vi "pid.vi"(7 "reset":bool, 8 "PID gains":T1, 9 "Enable motors":bool, 10 "Speed":cluster{"Left":dbl, "right":dbl}, 11 "Refnum in":refnum<k20>) -> (1 "output Speed":cluster{dbl, dbl}, 3 "Refnum out":refnum<k20>, 4 "dt out (s)":dbl format="%.3f")   [LabVIEW 2019]
uses:
  <vilib>/addons/control/pid/pid.llb/PID (DBL).vi
  <vilib>/Utility/error.llb/Error Cluster From Error Code.vi
  <vilib>/rvi/errors/niLvFpgaAdjustHostInterfaceError.vi
  <vilib>/rvi/interface/nirviReadWriteControl/nirviReadWriteControl.xnode
  NiFpgaLv.dll
  <vilib>/rvi/interface/Simulation/niFpgaSimulationCallBeginRW.vi
  <vilib>/addons/control/pid/NI_PID_pid.lvlib
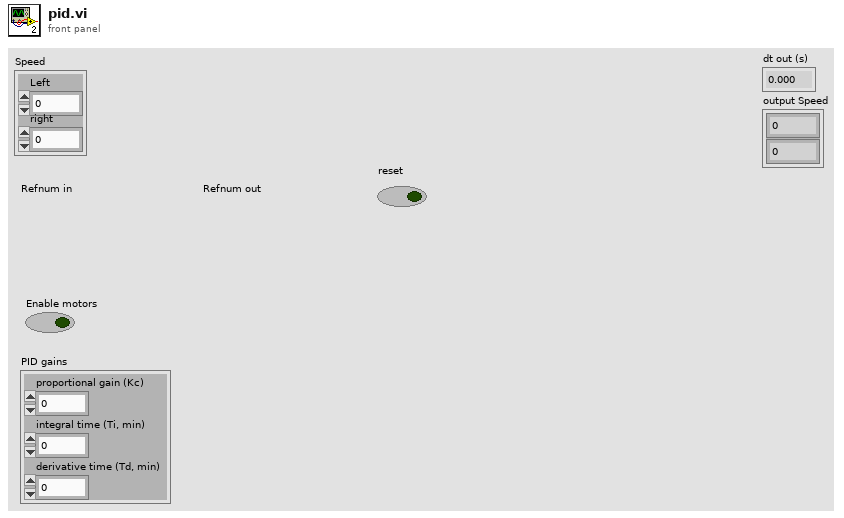
[diagram p1: front panel]
types:
  T1 = cluster{"proportional gain (Kc)":dbl, "integral time (Ti, min)":dbl, "derivative time (Td, min)":dbl}
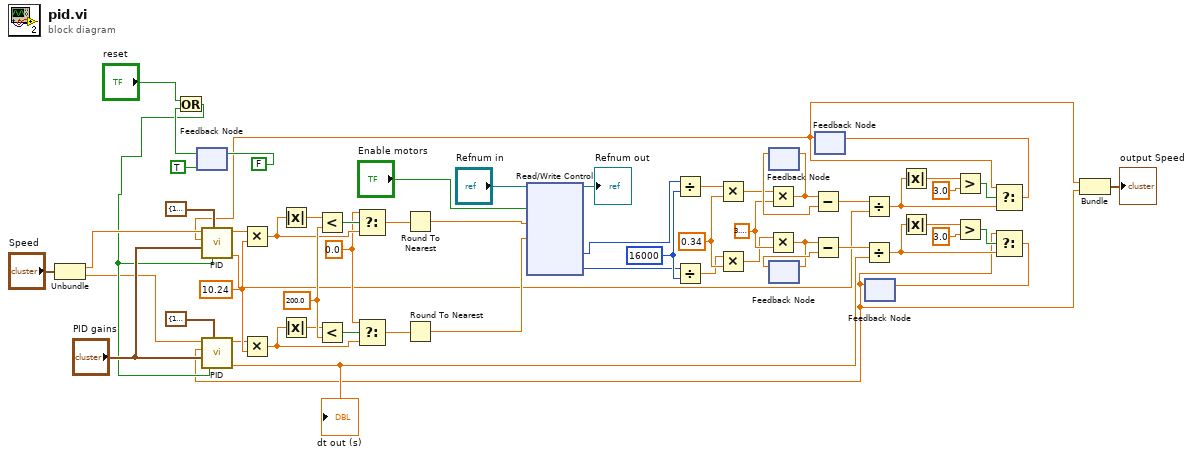
[diagram p0: block diagram]
diagram:
  w54 = 200.0 ("y")
  w47 = 0.0 ("t")
  w44 = 10.24 ("y")
  w26 = 3.141592653589793
  w23 = 0.34
  w20 = i64 16000 ("y")
  n1 = Unbundle("Speed") -> ("Left"=w9:dbl, "right"=w2:dbl)
  n2 = feedback #1(TRUE) -> (w5:bool)
  n3 = Or(x="reset", y=w5) -> (x .or. y?=w3:bool)
  n4 = feedback-in #1(FALSE) -> ()
  n5 = feedback #2() -> (w30:dbl)  [unwired: 1 in]
  n6 = feedback #3() -> (w28:dbl)  [unwired: 1 in]
  n7 = feedback #4() -> (w7:dbl)  [unwired: 1 in]
  n8 = call-poly <vilib>:"PID.vi"("reinitialize? (F)"=w3, "output range"=cluster{"output high":dbl, "output low":dbl} {"output high"=100.0, "output low"=-100.0}, "PID gains"="PID gains", "process variable"=w7, "setpoint"=w9) -> ("dt out (s)"=w10:dbl, "output"=w42:dbl)  [unwired: 5 in]
  n9 = Multiply(x=w42, y=w44) -> (x*y=w48:dbl)
  n10 = Absolute Value(x=w48) -> (abs(x)=w52:dbl)
  n11 = Less?(x=w52, y=w54) -> (x < y?=w50:bool)
  n12 = Select(t=w47, s=w50, f=w48) -> (s? t:f=w45:dbl)
  n13 = Round To Nearest(number=w45) -> (nearest integer value=w35:dbl)
  n14 = feedback #5() -> (w1:dbl)  [unwired: 1 in]
  n15 = call-poly <vilib>:"PID.vi"("reinitialize? (F)"=w3, "output range"=cluster{"output high":dbl, "output low":dbl} {"output high"=100.0, "output low"=-100.0}, "PID gains"="PID gains", "process variable"=w1, "setpoint"=w2) -> ("dt out (s)"=w12:dbl, "output"=w43:dbl)  [unwired: 5 in]
  "dt out (s)" <- w12
  n16 = Multiply(x=w43, y=w44) -> (x*y=w49:dbl)
  n17 = Absolute Value(x=w49) -> (abs(x)=w53:dbl)
  n18 = Less?(x=w53, y=w54) -> (x < y?=w51:bool)
  n19 = Select(t=w47, s=w51, f=w49) -> (s? t:f=w46:dbl)
  n20 = Round To Nearest(number=w46) -> (nearest integer value=w41:dbl)
  n21 = xnode "Read/Write Control"("FPGA VI Reference In"="Refnum in", "Motors"="Enable motors", "Left"=w35, "Right"=w41) -> ("FPGA VI Reference Out"=→"Refnum out":refnum<k20>, "Left"=w18:i64, "Right"=w19:i64)  [unwired: 1 in, 1 out]
  n22 = Divide(x=w18, y=w20) -> (x/y=w21:dbl)
  n23 = Divide(x=w19, y=w20) -> (x/y=w22:dbl)
  n24 = Multiply(x=w21, y=w23) -> (x*y=w24:dbl)
  n25 = Multiply(x=w22, y=w23) -> (x*y=w25:dbl)
  n26 = Multiply(x=w24, y=w26) -> (x*y=w29:dbl)
  n27 = Multiply(x=w25, y=w26) -> (x*y=w27:dbl)
  n28 = feedback-in #2(w29) -> ()
  n29 = feedback-in #3(w27) -> ()
  n30 = Subtract(x=w29, y=w30) -> (x-y=w31:dbl)
  n31 = Subtract(x=w27, y=w28) -> (x-y=w32:dbl)
  n32 = Divide(x=w31, y=w10) -> (x/y=w15:dbl)
  n33 = Divide(x=w32, y=w12) -> (x/y=w14:dbl)
  n34 = Absolute Value(x=w15) -> (abs(x)=w38:dbl)
  n35 = Absolute Value(x=w14) -> (abs(x)=w57:dbl)
  n36 = Greater?(x=w38, y=3.0) -> (0:w39:bool)
  n37 = Greater?(x=w57, y=3.0) -> (0:w58:bool)
  n38 = Select(t=w7, s=w39, f=w15) -> (s? t:f=w11:dbl)
  n39 = feedback-in #4(w11) -> ()
  n40 = Select(t=w1, s=w58, f=w14) -> (s? t:f=w13:dbl)
  n41 = feedback-in #5(w13) -> ()
  n42 = Bundle(w7, w1) -> (→"output Speed":cluster{dbl, dbl})  [unwired: 1 in]
